vi "subsystem_acceptCommand_Disable.vi"(8 "error in (no error)":errorcluster, 11 "ProgrammaticInitialization in":refnum<class "ProgrammaticInitialization.lvclass">) -> (0 "error out":errorcluster, 1 "function return":i32, 2 "command_Disable":T1, 3 "ProgrammaticInitialization out":refnum<class "ProgrammaticInitialization.lvclass">)   [LabVIEW 2016, in "ProgrammaticInitialization.lvclass"]
uses:
  ProgrammaticInitialization.lvclass
  ts_sallv_sedspectrometer/DataTypes/command_disable.ctl
  commandType.ctl
  ProgrammaticInitialization.lvclass/ProgrammaticInitialization.ctl
  ts_sallv_sedspectrometer/SALLV_sedSpectrometer.lvlib
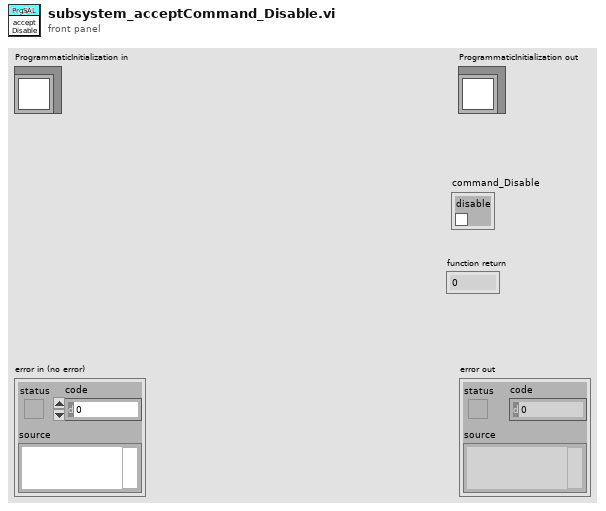
[diagram p1: front panel]
types:
  T1 = typedef "SALLV_sedSpectrometer.lvlib/command_disable.ctl" = cluster{"disable":bool}
  T2 = typedef "ProgrammaticInitialization.lvclass/commandType.ctl" = enum16{"acceptCommand", "ackCommand", "cancelCallback_command", "cancelCallback_logEvent", "cancelCallback", "flushSamplesEvent", "getEvent", "getNextSample", "getResponse", "getSample", "issueCommand", "logEvent", "monitorCommand", "putSample", "registerCallback_command", "registerCallback_logEvent", "registerCallback", "salCommander", "salEvent", "salProcessor", "salTelemetrySub", "waitForCompletion"}
  T3 = typedef "SALLV_EXA.lvlib/command_Disable.ctl" = cluster{"disable":bool}
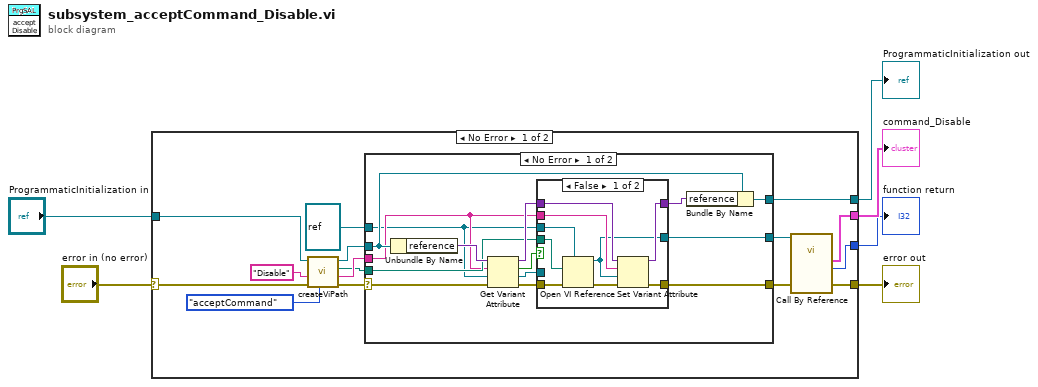
[diagram p0: block diagram]
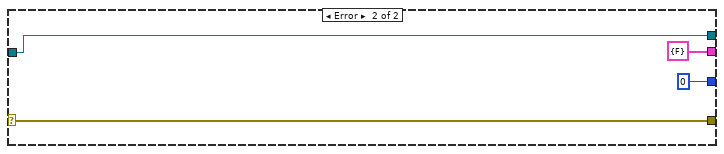
[diagram p4: hidden frame]
diagram:
  n1 = case shown="No Error" "error in (no error)" {
    selector: "error in (no error)" -> [w19 w54]
    tunnel: [w16 w54] -> w5
    tunnel: [w13 w53] -> w3
    tunnel: "ProgrammaticInitialization in" -> [w14 w53]
    tunnel: [w18 T1 {"disable"=FALSE} ("command_Disable_Ctl out")] -> w2
    tunnel: [w17 0 ("function return")] -> w1
    frame No Error {
      n2 = call "createViPath.vi"("CommandType"=commandType."acceptCommand", "error in (no error)"=w19, "topic"="Disable", "ProgrammaticInitialization in"=w14) -> ("error out"=w12:errorcluster, "vi name"=w11:string, "path"=w10:path, "ProgrammaticInitialization out"=w15:refnum<class "ProgrammaticInitialization.lvclass">)  [unwired: 4 in]
      n3 = case shown="No Error" w12 {
        selector: w12 -> [w32 w50]
        tunnel: [w31 w50] -> w7
        tunnel: [w27 w49] -> w13
        tunnel: w15 -> [w26 w49]
        tunnel: w11 -> [w24 _]
        tunnel: refnum<vi> refnum ("type specifier VI Refnum (for type only)") -> [w22 w48]
        tunnel: w10 -> [w25 _]
        tunnel: [w23 w48] -> w8
        frame No Error {
          n4 = Unbundle By Name(w26) -> ("reference"=w30:variant)
          n5 = Get Variant Attribute(Variant=w30, name=w24, default value (empty Variant)=w22, error in=w32) -> (duplicate Variant=w29:variant, found=w35:bool, value=w33:refnum<vi>, error out=w34:errorcluster)
          n6 = case shown="False" w35 {
            tunnel: w34 -> [w42 w47]
            tunnel: w33 -> [_ w45]
            tunnel: [w44 w47] -> w31
            tunnel: w29 -> [w37 w46]
            tunnel: [w43 w46] -> w28
            tunnel: w22 -> [w40 _]
            tunnel: w25 -> [w39 _]
            tunnel: w24 -> [w38 _]
            tunnel: [w36 w45] -> w23
            frame False {
              n7 = Open VI Reference(type specifier VI Refnum (for type only)=w40, vi path=w39, error in (no error)=w42) -> (vi reference=w36:refnum<vi>, error out=w41:errorcluster)  [unwired: 3 in]
              n8 = Set Variant Attribute(Variant=w37, name=w38, value=w36, error in=w41) -> (Variant out=w43:variant, error out=w44:errorcluster)  [unwired: 1 out]
            }
            frame True {
            }
          }
          n9 = Bundle By Name(cluster=w26, "reference"=w28) -> (w27:refnum<class "ProgrammaticInitialization.lvclass">)
        }
        frame Error {
        }
      }
      n10 = call-by-ref "?"(reference=w8, "error in (no error)"=w7) -> ("error out"=w16:errorcluster, "function return"=w17:i32, "command_Disable_Ctl out"=w18:T3)  [unwired: 9 in, 2 out]
    }
    frame Error {
    }
  }
  "error out" <- w5
  "ProgrammaticInitialization out" <- w3
  "command_Disable" <- w2
  "function return" <- w1
